vi "GetEncoderValues.vi"(8 "error in":errorcluster) -> (0 "error out":errorcluster, 2 "RightDistance":dbl, 3 "LeftDistance":dbl)   [LabVIEW 2016]
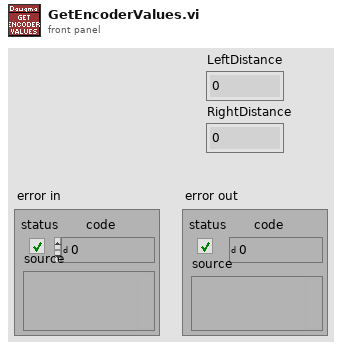
[diagram p1: front panel]
types:
  T1 = typedef "WPI_EncoderDevRef.ctl" = cluster{"DevStatus":errorcluster, "EncoderIndex":T2, "CounterIndex":T3, "DistancePerCount":dbl, "Decoding Type":T4}
  T2 = typedef "FPGA_EncoderIdx.ctl" = enum8{"Enc 0", "Enc 1", "Enc 2", "Enc 3", "Enc 4", "Enc 5", "Enc 6", "Enc 7", "Invalid"}
  T3 = typedef "FPGA_CounterCtrSystemIndex.ctl" = enum8{"Ctr 0", "Ctr 1", "Ctr 2", "Ctr 3", "Ctr 4", "Ctr 5", "Ctr 6", "Ctr 7", "Invalid"}
  T4 = typedef "WPI_EncoderType.ctl" = enum16{"1x", "2x", "4x"}
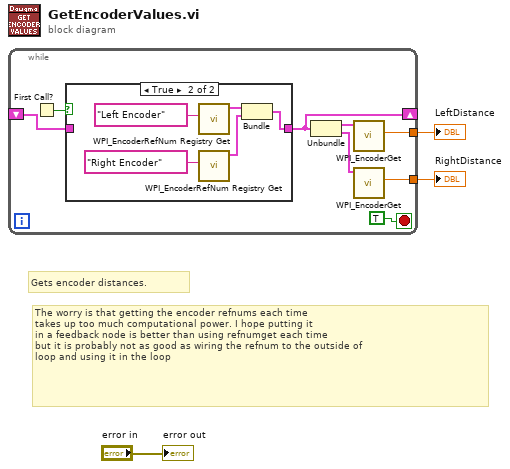
[diagram p0: block diagram]
diagram:
  # "The worry is that getting the encoder refnums each time\ntakes up too much computational power. I hope putting it\nin a feedback node is better than using refnumget each time\nbut it is probably not as good as wiring the refnum to the outside of\nloop and using it in the loop"
  # "Gets encoder distances."
  n1 = while {
    shift-right: [w8] -> _
    shift-left: _ -> [w9]
    tunnel: [w5] -> w3
    tunnel: [w4] -> w2
    stop <- TRUE stop-if-true
    n2 = First Call?() -> (First Call?: T/F=w10:bool)
    n3 = case shown="True" w10 {
      tunnel: [w12 w13] -> w8
      tunnel: w9 -> [w12 _]
      frame False {
      }
      frame True {
        n4 = call <vilib>:"WPI_EncoderRefNum Registry Get.vi"("refnum name"="Left Encoder") -> ("EncoderDevRef"=w15:T1)  [unwired: 9 in, 1 out]
        n5 = call <vilib>:"WPI_EncoderRefNum Registry Get.vi"("refnum name"="Right Encoder") -> ("EncoderDevRef"=w14:T1)  [unwired: 9 in, 1 out]
        n6 = Bundle("EncoderDevRef"=w15, "EncoderDevRef"=w14) -> (w13:cluster{"EncoderDevRef":T1, "EncoderDevRef":T1})  [unwired: 1 in]
      }
    }
    n7 = Unbundle(w8) -> ("EncoderDevRef"=w7:T1, "EncoderDevRef"=w6:T1)
    n8 = call <vilib>:"WPI_EncoderGet.vi"("EncoderDevRef"=w7) -> ("Distance"=w5:dbl)  [unwired: 5 in, 5 out]
    n9 = call <vilib>:"WPI_EncoderGet.vi"("EncoderDevRef"=w6) -> ("Distance"=w4:dbl)  [unwired: 5 in, 5 out]
  }
  "LeftDistance" <- w3
  "RightDistance" <- w2
  "error out" <- "error in"
